vi "Read LVDT's Data.vi"(5 "Desired Decimal Points":u8=2, 7 "truncate instead of round":bool, 8 "error in":errorcluster, 9 "LVDT's Limits":T1[](array[typedef]) {"Lower Limit" format="%.2f"; "Upper Limit" format="%.2f"}, 10 "rs232?":bool=TRUE, 11 "LVDT's Com Port":refnum<visa-resource-name>="COM6") -> (0 "error out":errorcluster, 3 "Array":sgl[](array[numeric]))   [LabVIEW 2018]
uses:
  type defs/EOL LVDT's Check Controller.ctl
  <vilib>/Instr/_visa.llb/VISA Configure Serial Port (Instr).vi
panel:
  in  "LVDT Unit 1 ip":string
  out "read buffer":string
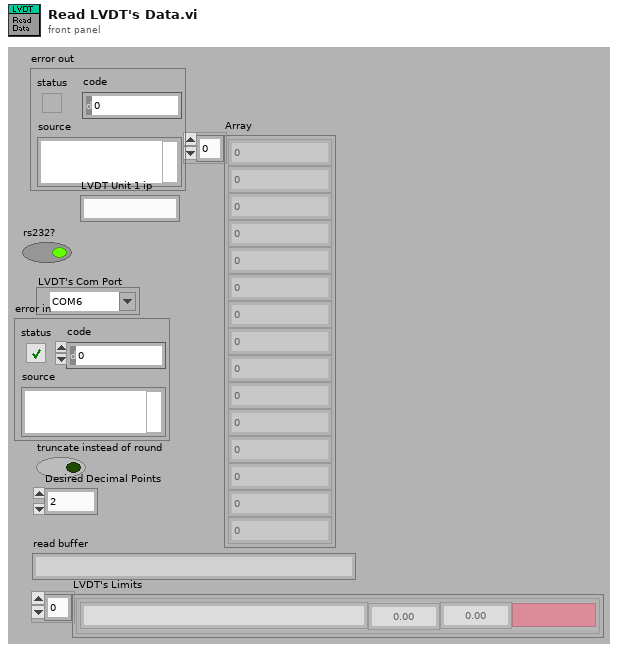
[diagram p1: front panel]
types:
  T1 = typedef "EOL LVDT's Check Controller.ctl" = cluster{"Upper Limit":dbl, "Lower Limit":dbl, "LVDT Name":string, "Check":bool}
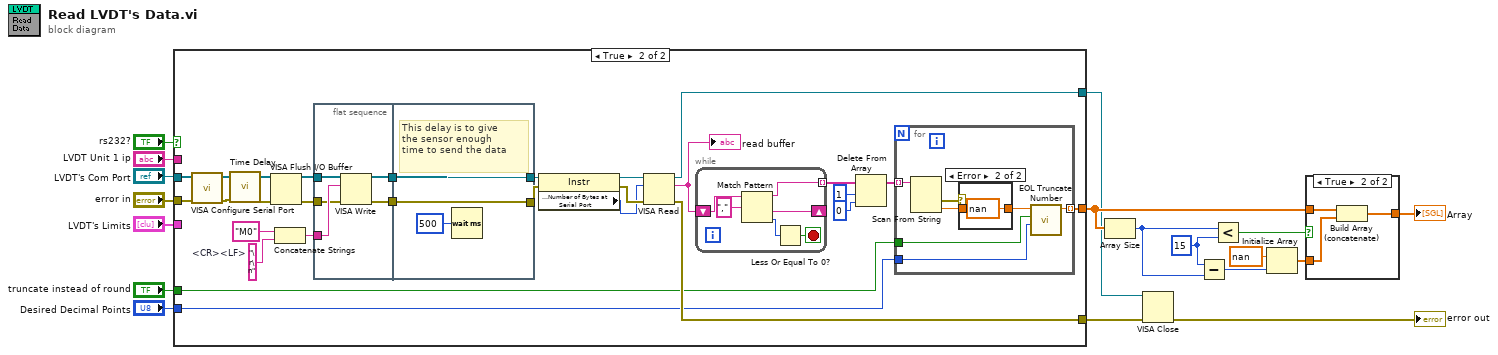
[diagram p0: block diagram]
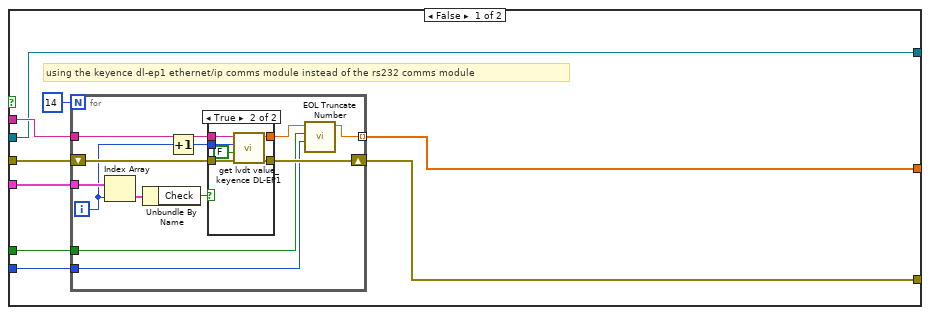
[diagram p2: hidden frame]
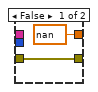
[diagram p3: hidden frame]
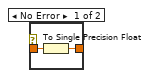
[diagram p4: hidden frame]
diagram:
  w14 = 15 ("y")
  n1 = case shown="True" "rs232?" {
    tunnel: [w22 w70] -> w12
    tunnel: "LVDT's Com Port" -> [w19 w51]
    tunnel: [w23 w68] -> w2
    tunnel: "error in" -> [w25 w53]
    tunnel: "truncate instead of round" -> [w21 w67]
    tunnel: "Desired Decimal Points" -> [w20 w66]
    tunnel: "LVDT Unit 1 ip" -> [w26 _]
    tunnel: "LVDT's Limits" -> [w24 _]
    tunnel: [w19 w48] -> w3
    frame False {
      # "using the keyence dl-ep1 ethernet/ip comms module instead of the rs232 comms module"
      n2 = for {
        N: 14 -> [_]
        tunnel: w26 -> [w37]
        shift-right: [w38] -> w23
        shift-left: w25 -> [w39]
        tunnel: w24 -> [w36]
        tunnel: [w30] -> w22 mode=indexing
        tunnel: w21 -> [w29]
        tunnel: w20 -> [w28]
        i -> [w34]
        n3 = Index Array(array=w36, index=w34) -> (element=w35:T1)
        n4 = Unbundle By Name(w35) -> ("Check"=w32:bool)
        n5 = Increment(x=w34) -> (x+1=w33:i32)
        n6 = case shown="True" w32 {
          tunnel: w39 -> [w41 w47]
          tunnel: [w41 w46] -> w38
          tunnel: w37 -> [_ w44]
          tunnel: w33 -> [_ w43]
          tunnel: [nan ("PV") w42] -> w31
          frame False {
          }
          frame True {
            n7 = call "get lvdt value_keyence DL-EP1.vi"("error in"=w47, "update preset"=FALSE, "Instance ID in  (LVDT Amplifier Index [1..n])"=w43, "Network Path"=w44) -> ("error out"=w46:errorcluster, "PV"=w42:dbl)  [unwired: 5 in, 1 out]
          }
        }
        n8 = call "EOL Truncate Number.vi"("Desired Decimal Points"=w28, "truncate instead of round"=w29, "Numeric Input"=w31) -> ("Numeric Output"=w30:sgl)  [unwired: 8 in]
      }
    }
    frame True {
      w57 = "\r\n"  # <CR><LF>
      n9 = call-poly "VISA Configure Serial Port"("VISA resource name"=w51, "error in (no error)"=w53) -> ("VISA resource name out"=w50:refnum<visa-resource-name>, "error out"=w52:errorcluster)  [unwired: 12 in]
      n10 = call "Time Delay"("error in (no error)"=w52) -> ("error out"=w49:errorcluster)  [unwired: 10 in]
      n11 = VISA Flush I/O Buffer(VISA resource name=w50, error in (no error)=w49) -> (VISA resource name out=w59:refnum<visa-resource-name>, error out=w60:errorcluster)  [unwired: 1 in]
      n12 = Concatenate Strings("M0" ("write buffer"), w57) -> (w58:string)
      n13 = flat-sequence {
        tunnel: w59 -> [w79]
        tunnel: w58 -> [w78]
        tunnel: [w77] -> w62
        tunnel: w60 -> [w76]
        tunnel: [w75] -> w61
        tunnel: w62 -> [w82]
        tunnel: [w82] -> w54
        tunnel: [w81] -> w55
        tunnel: w61 -> [w81]
        frame #0 {
          n14 = VISA Write(VISA resource name=w79, write buffer=w78, error in (no error)=w76) -> (VISA resource name out=w77:refnum<visa-resource-name>, error out=w75:errorcluster)  [unwired: 1 out]
        }
        frame #1 {
          # "This delay is to give\nthe sensor enough\ntime to send the data"
          n15 = Wait (ms)(milliseconds to wait=u32 500) -> ()  [unwired: 1 out]
        }
      }
      n16 = property class="Instr"(reference=w54, error in=w55) -> (reference out=w65:refnum<visa-resource-name>, error out=w64:errorcluster, "Serial Settings:Number of Bytes at Serial Port"=w63:u32)
      n17 = VISA Read(VISA resource name=w65, byte count=w63, error in (no error)=w64) -> (VISA resource name out=w48:refnum<visa-resource-name>, read buffer=w69:string, error out=w68:errorcluster)  [unwired: 1 out]
      "read buffer" <- w69
      n18 = while {
        tunnel: [w94] -> w74 mode=indexing
        shift-right: [w96] -> _
        shift-left: w69 -> [w98]
        stop <- w95 stop-if-true
        n19 = Match Pattern(string=w98, regular expression=",") -> (before substring=w94:string, after substring=w96:string, offset past match=w93:i32)  [unwired: 1 in, 1 out]
        n20 = Less Or Equal To 0?(x=w93) -> (x <= 0?=w95:bool)
      }
      n21 = Delete From Array(array=w74, length=1, index=0) -> (array with subset deleted=w71:string[])  [unwired: 1 out]
      n22 = for {
        tunnel: w71 -> [w89] mode=indexing
        tunnel: [w85] -> w70 mode=indexing
        tunnel: w67 -> [w84]
        tunnel: w66 -> [w83]
        n23 = Scan From String(input string=w89) -> (error out=w88:errorcluster, output 1=w87:dbl)  [unwired: 4 in, 2 out]
        n24 = case shown="Error" w88 {
          tunnel: w87 -> [w91 _]
          tunnel: [w90 sgl nan] -> w86
          frame No Error {
            n25 = To Single Precision Float(number=w91) -> (single precision float=w90:sgl)
          }
          frame Error {
          }
        }
        n26 = call "EOL Truncate Number.vi"("Desired Decimal Points"=w83, "truncate instead of round"=w84, "Numeric Input"=w86) -> ("Numeric Output"=w85:sgl)  [unwired: 8 in]
      }
    }
  }
  n27 = Array Size(array=w12) -> (size(s)=w16:i32)
  n28 = VISA Close(VISA resource name=w3, error in (no error)=w2) -> (error out=→"error out":errorcluster)
  n29 = Subtract(x=w14, y=w16) -> (x-y=w18:i32)
  n30 = Less?(x=w16, y=w14) -> (x < y?=w15:bool)
  n31 = Initialize Array(sgl nan ("element"), w18) -> (w13:sgl[])
  n32 = case shown="True" w15 {
    tunnel: w12 -> [w99 w102]
    tunnel: w13 -> [_ w101]
    tunnel: [w99 w100] -> w11
    frame False {
    }
    frame True {
      n33 = Build Array (concatenate)(w102, w101) -> (w100:sgl[])
    }
  }
  "Array" <- w11
